vi "better_autoscale_z.vi"(1 "Input Array":i32[][](array[numeric])) -> (0 "autoscale max":dbl)   [LabVIEW 2013]
panel:
  out "array average":dbl
  out "Intensity Graph":dbl[][](graph)
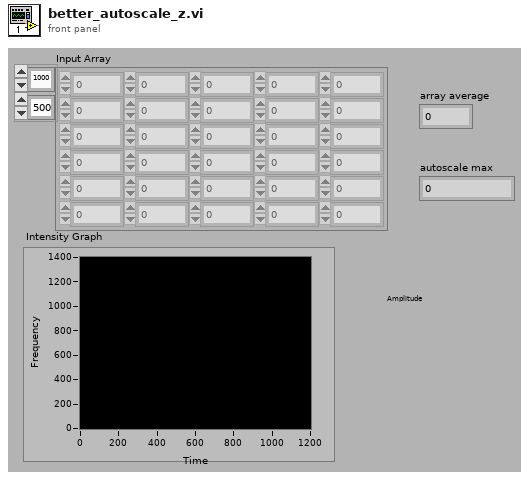
[diagram p1: front panel]
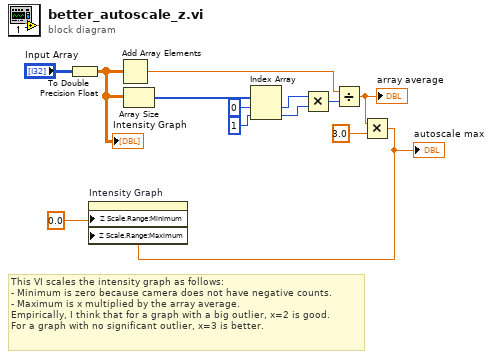
[diagram p0: block diagram]
diagram:
  # "This VI scales the intensity graph as follows:\n- Minimum is zero because camera does not have negative counts.\n- Maximum is x multiplied by the array average.\nEmpirically, I think that for a graph with a big outlier, x=2 is good.\nFor a graph with no significant outlier, x=3 is better."
  n1 = To Double Precision Float(number="Input Array") -> (double precision float=w1:dbl[][])
  "Intensity Graph" <- w1
  n2 = Add Array Elements(numeric array=w1) -> (sum=w6:dbl)
  n3 = Array Size(array=w1) -> (size(s)=w12:i32[])
  n4 = Index Array(array=w12, index #1=0 ("index"), index #2=1 ("index")) -> (element #1=w9:i32, element #2=w8:i32)
  n5 = Multiply(x=w9, y=w8) -> (x*y=w7:i32)
  n6 = Divide(x=w6, y=w7) -> (x/y=w5:dbl)
  "array average" <- w5
  n7 = Multiply(x=w5, y=3.0) -> (x*y=w3:dbl)
  "autoscale max" <- w3
  n8 = property on="Intensity Graph" class="IntGraph (strict)"("Z Scale.Range:Minimum"=0.0, "Z Scale.Range:Maximum"=w3) -> ()  [unwired: 2 in, 2 out]
